vi "Copy Packaging Components.vi"(0 "Primary destination path":path, 5 "Template Path":path, 11 "error in (no error)":errorcluster) -> (4 "Package Files":path[](array[path]), 15 "error out":errorcluster)   [LabVIEW 2021, in "Packager Helpers.lvlib"]
uses:
  Packager Helpers.lvlib
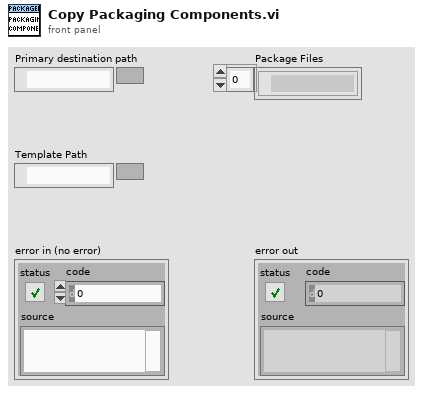
[diagram p1: front panel]
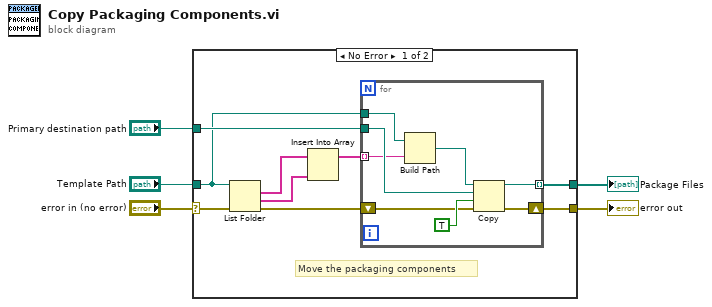
[diagram p0: block diagram]
diagram:
  n1 = case shown="No Error" "error in (no error)" {
    selector: "error in (no error)" -> [w9 w23]
    tunnel: "Template Path" -> [w11 _]
    tunnel: [w7 w23] -> w4
    tunnel: "Primary destination path" -> [w12 _]
    tunnel: [w6 _] -> w1
    frame No Error {
      # "Move the packaging components"
      n2 = List Folder(path=w11, error in=w9) -> (filenames=w13:string[], folder names=w14:string[], error out=w8:errorcluster)  [unwired: 2 in, 1 out]
      n3 = Insert Into Array(array=w13, new element=w14) -> (w10:string[])  [unwired: 1 in]
      n4 = for {
        shift-right: [w17] -> w7
        shift-left: w8 -> [w18]
        tunnel: w10 -> [w15] mode=indexing
        tunnel: w12 -> [w20]
        tunnel: w11 -> [w19]
        tunnel: [w16] -> w6 mode=indexing
        n5 = Build Path(base path=w19, name or relative path=w15) -> (appended path=w22:path)
        n6 = Copy(8:w18, 9:TRUE ("overwrite (F)"), 10:w20, 11:w22) -> (0:w17:errorcluster, 3:w16:path)  [unwired: 1 in, 1 out]
      }
    }
    frame Error {
    }
  }
  "error out" <- w4
  "Package Files" <- w1
